vi "Cleanup.vi"(8 "error in (no error)":errorcluster, 9 "Module Routes":refnum<user-event>[](array[refnum]), 11 "Event Refs":refnum<event-registration>[](array[refnum])) -> (0 "error out":errorcluster)   [LabVIEW 2016]
doc: "Cleanup references from the application"
uses:
  Message Queue/Message Cluster.ctl
  Message Queue/Message Queue.lvlib
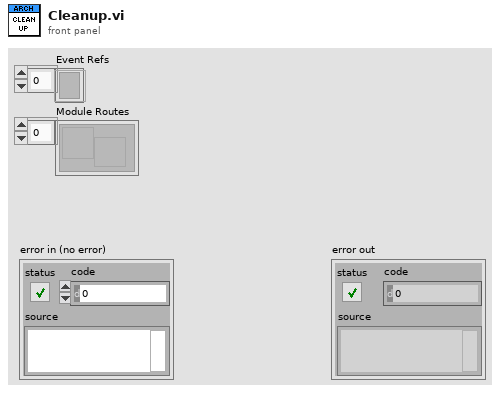
[diagram p1: front panel]
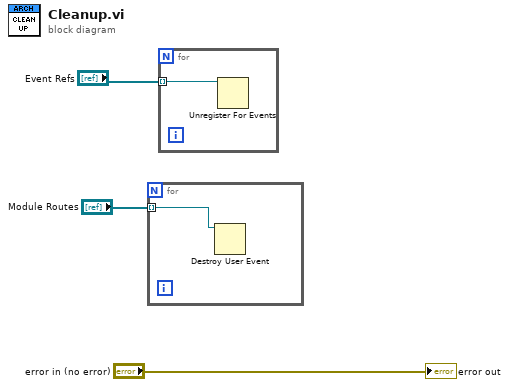
[diagram p0: block diagram]
diagram:
  n1 = for {
    tunnel: "Module Routes" -> [w4] mode=indexing
    n2 = Destroy User Event(user event=w4) -> ()  [unwired: 1 in, 1 out]
  }
  n3 = for {
    tunnel: "Event Refs" -> [w5] mode=indexing
    n4 = Unregister For Events(event registration refnum=w5) -> ()  [unwired: 1 in, 1 out]
  }
  "error out" <- "error in (no error)"
